vi "OneCode.vi"(9 "VI Name":string, 11 "Default":T1) -> ()   [LabVIEW 2016]
uses:
  VIs/uPythonX/uPythonX.xctl
panel:
  in  "main.py":T1(xcontrol)
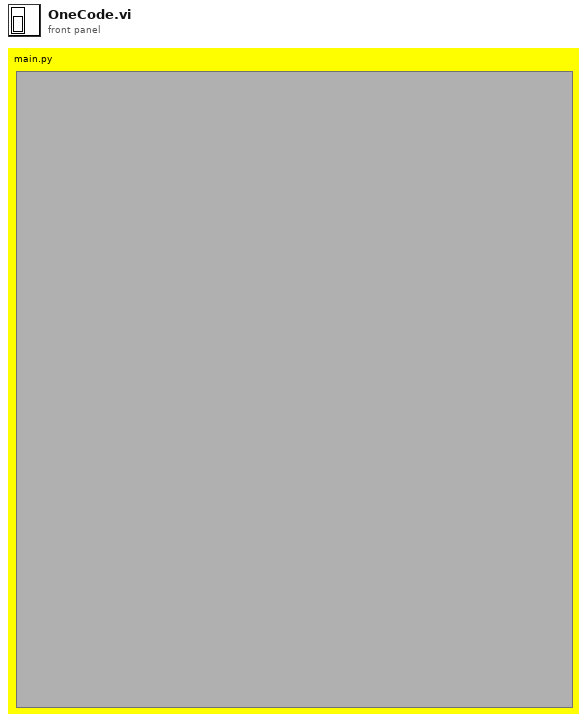
[diagram p1: front panel]
types:
  T1 = cluster{"Port":refnum<visa-resource-name>, "All Code":string}
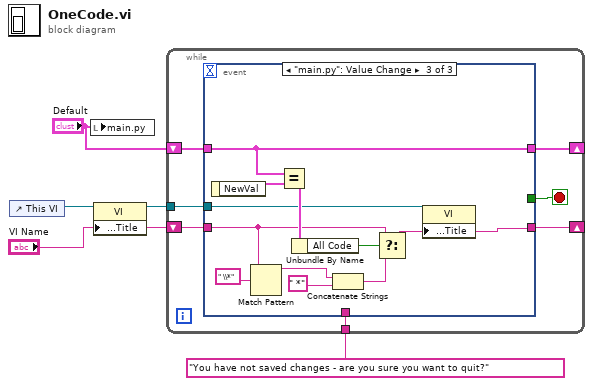
[diagram p0: block diagram]
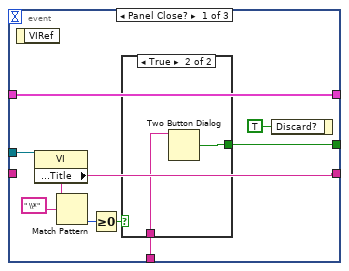
[diagram p2: hidden frame]
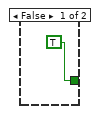
[diagram p3: hidden frame]
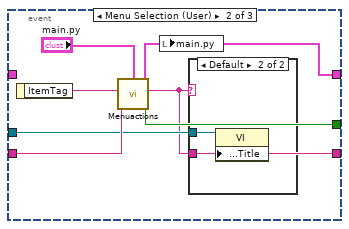
[diagram p4: hidden frame]
diagram:
  n1 = control-ref of="This VI"() -> (w5:refnum<vi>)
  n2 = local write "main.py"("Default") -> ()
  n3 = property class="VI"(reference=w5, "Front Panel.Title"="VI Name") -> (reference out=w4:refnum<vi>)  [unwired: 1 in, 1 out]
  n4 = while {
    tunnel: w4 -> [w11]
    shift-right: [w9] -> _
    shift-left: "VI Name" -> [w10]
    shift-right: [w7] -> _
    shift-left: "Default" -> [w8]
    tunnel: "You have not saved changes - are you sure you want to quit?" ("message") -> [w6]
    stop <- w12 stop-if-true
    n5 = event shown="[2] \"main.py\": Value Change" {
      selector: _ -> [_ _ _]
      dyn-events: _ -> [_ _ _]
      timeout: _ -> [_ _ _]
      tunnel: [w16 w29 _] -> w12
      tunnel: w11 -> [w21 w28 w42]
      tunnel: w10 -> [_ w30 w35]
      tunnel: [w20 w27 w39] -> w9
      tunnel: w8 -> [w15 _ w37]
      tunnel: [w15 w25 w37] -> w7
      tunnel: w6 -> [w13 _ _]
      event Panel Close? {
        n6 = event-data() -> ()  [unwired: 1 in, 1 out]
        n7 = property class="VI"(reference=w21) -> ("Front Panel.Title"=w20:string)  [unwired: 1 in, 2 out]
        n8 = Match Pattern(string=w20, regular expression=" \\*" ("string")) -> (offset past match=w19:i32)  [unwired: 1 in, 3 out]
        n9 = Greater Or Equal To 0?(x=w19) -> (x >= 0?=w18:bool)
        n10 = case shown="True" w18 {
          tunnel: [TRUE ("T button?") w24] -> w16
          tunnel: w13 -> [_ w23]
          frame False {
          }
          frame True {
            n11 = Two Button Dialog(message=w23) -> (T button?=w24:bool)  [unwired: 2 in]
          }
        }
        n12 = event-data("Discard?"=TRUE) -> ()  [unwired: 1 in, 1 out]
      }
      event Menu Selection (User) {
        n13 = event-data() -> ("ItemTag"=w31:string)  [unwired: 1 in]
        n14 = call "Menuactions.vi"("Name"=w30, "ItemTag"=w31, "Default in"="main.py") -> ("Close?"=w29:bool, "Name out"=w27:string, "Default out"=w25:T1)  [unwired: 6 in]
        n15 = local write "main.py"(w25) -> ()
        n16 = case shown="Default" w27 {
          tunnel: w28 -> [_ w33]
          tunnel: w27 -> [_ w32]
          frame "" {
          }
          frame Default {
            n17 = property class="VI"(reference=w33, "Front Panel.Title"=w32) -> ()  [unwired: 1 in, 2 out]
          }
        }
      }
      event "main.py": Value Change {
        n18 = event-data() -> ("NewVal"=w38:T1)  [unwired: 1 in]
        n19 = Match Pattern(string=w35, regular expression=" \\*" ("string")) -> (before substring=w34:string)  [unwired: 1 in, 3 out]
        n20 = Equal?(x=w37, y=w38) -> (x = y?=w44:cluster{"Port":bool, "All Code":bool})
        n21 = Unbundle By Name(w44) -> ("All Code"=w43:bool)
        n22 = Concatenate Strings(w34, " *" ("string")) -> (w41:string)
        n23 = Select(t=w35, s=w43, f=w41) -> (s? t:f=w39:string)
        n24 = property class="VI"(reference=w42, "Front Panel.Title"=w39) -> ()  [unwired: 1 in, 2 out]
      }
    }
  }
